vi "AlliGator Get-Set Loading & Pre-Processing Options.vi"(6 "Get (F)/Set":bool, 8 "Error In":errorcluster, 11 "Dataset Loading & Pre-processing Options (in)":T1={"Data Information"={"Gates to Skip"={"Start"=0, "End"=0}, "# Gates"=1, "Gate Step"=1, "Gate Duration"=3e-10, "Gate Separation"=4e-11, "Pile-up Correction"=FALSE, "Pixel Well Capacity"=1, "Define Gates to"=enum."Skip", "Gates to Keep"={"First"=0, "Last"=0}, "Laser Period"=0.0, "SYNC Period"=0.0, "Channel Name"=0, "Channel Arithmetic"=enum."None", "Background File Subtraction"=FALSE, "Background Scaling Factor"=1.0, "Background File"=path "", "Background Pile-up Correction"=FALSE, "Background Pixel Well Capacity"=1, "Dataset Scaling Factor"=1.0}, "Source Image Settings"={"Low Count Pixels Rejection Options"={"Background Low Threshold Factor"=0.0, "Fixed Low Background Threshold"=20000.0, "Reject Low Count Pixels"=FALSE, "Low Percentile"=0.0}, "High Count Pixels Rejection Options"={"Background High Threshold Factor"=0.0, "Fixed High Background Threshold"=1.0, "Reject High Count Pixels"=FALSE, "High Percentile"=100.0}, "Peak Threshold"=500.0, "Intensity Threshold"=500.0, "Image Smoothing Options"={"Use Image Smoothing"=FALSE, "Kernel Type"=enum."Bilinear", "Bin"=1, "Algorithm"=enum."Rapid"}, "Image Binning Options"={"Use Image Binning"=FALSE, "X Bin"=1, "Y Bin"=1}}, "Decay Preprocessing Options & Parameters"={"Background Subtraction Parameters"={"Background Definition Range"={"Min Gate"=0.0, "Max Gate"=0.0}, "Baseline Subtraction Method"=enum."Mean", "Background Subtraction?"=FALSE, "Background File"=path "", "Background Constant"=0.0, "Background Scaling Factor"=1.0, "Background Pile-up Correction"=FALSE, "Background Pixel Well Capacity"=1}, "Decay Preprocessing Parameters"={"Background Subtraction"=FALSE, "Straighten Decay"=FALSE, "Reverse Gates"=FALSE, "1-Normalized Decay"=FALSE, "Smoothen Decay"=FALSE, "Smoothing Parameter"=0.0, "Shift Decay"=FALSE, "Decay Shift Parameters"={"Type"=enum."Default", "Shift"=0.0, "Threshold"=0.0, "Rotate"=FALSE}, "Extrapolate Decay"=FALSE, "Additional Points"=0, "Head Fraction"=0.0, "Pixel-Normalize Decay"=FALSE, "Use Periodicity"=FALSE, "Use Cursors"=FALSE, "Tail Fraction"=0.0, "Use Decay Pre-Processing"=TRUE, "Fold Decay"=FALSE, "# Folds"=1, "[0-1]-Normalized Decay"=FALSE}, "Preprocessing Steps Order"=[]}, "Clear Phasor Graph"=FALSE} {"Decay Preprocessing Options & Parameters"."Decay Preprocessing Parameters"."# Folds" min=1; "Decay Preprocessing Options & Parameters"."Background Subtraction Parameters"."Background Pixel Well Capacity" min=1 step=1; "Source Image Settings"."Image Binning Options"."Y Bin" min=1; "Source Image Settings"."Image Binning Options"."X Bin" min=1; "Source Image Settings"."Image Smoothing Options"."Bin" min=1; "Source Image Settings"."High Count Pixels Rejection Options"."High Percentile" min=0.0 max=100.0; "Source Image Settings"."Low Count Pixels Rejection Options"."Low Percentile" min=0.0 max=100.0; "Data Information"."Background Pixel Well Capacity" min=1 step=1; "Data Information"."Channel Name" items=["Bottom INT Gate", "Bottom G2 Gate"]; "Data Information"."SYNC Period" min=0.0 format="%#.3g"; "Data Information"."Laser Period" min=0.0 format="%#.3g"; "Data Information"."Pixel Well Capacity" min=1 step=1; "Data Information"."# Gates" min=1 step=1; "Data Information"."Gate Step" min=1 step=1; "Data Information"."Gate Duration" min=0.0 format="%#.3g"; "Data Information"."Gate Separation" min=0.0 format="%#.3g"}) -> (0 "Error Out":errorcluster, 3 "Dataset Loading & Pre-processing Options (out)":T1={"Data Information"={"Gates to Skip"={"Start"=0, "End"=0}, "# Gates"=1, "Gate Step"=1, "Gate Duration"=3e-10, "Gate Separation"=4e-11, "Pile-up Correction"=FALSE, "Pixel Well Capacity"=1, "Define Gates to"=enum."Skip", "Gates to Keep"={"First"=0, "Last"=0}, "Laser Period"=0.0, "SYNC Period"=0.0, "Channel Name"=0, "Channel Arithmetic"=enum."None", "Background File Subtraction"=FALSE, "Background Scaling Factor"=1.0, "Background File"=path "", "Background Pile-up Correction"=FALSE, "Background Pixel Well Capacity"=1, "Dataset Scaling Factor"=1.0}, "Source Image Settings"={"Low Count Pixels Rejection Options"={"Background Low Threshold Factor"=0.0, "Fixed Low Background Threshold"=20000.0, "Reject Low Count Pixels"=FALSE, "Low Percentile"=0.0}, "High Count Pixels Rejection Options"={"Background High Threshold Factor"=0.0, "Fixed High Background Threshold"=1.0, "Reject High Count Pixels"=FALSE, "High Percentile"=100.0}, "Peak Threshold"=500.0, "Intensity Threshold"=500.0, "Image Smoothing Options"={"Use Image Smoothing"=FALSE, "Kernel Type"=enum."Bilinear", "Bin"=1, "Algorithm"=enum."Rapid"}, "Image Binning Options"={"Use Image Binning"=FALSE, "X Bin"=1, "Y Bin"=1}}, "Decay Preprocessing Options & Parameters"={"Background Subtraction Parameters"={"Background Definition Range"={"Min Gate"=0.0, "Max Gate"=0.0}, "Baseline Subtraction Method"=enum."Mean", "Background Subtraction?"=FALSE, "Background File"=path "", "Background Constant"=0.0, "Background Scaling Factor"=1.0, "Background Pile-up Correction"=FALSE, "Background Pixel Well Capacity"=1}, "Decay Preprocessing Parameters"={"Background Subtraction"=FALSE, "Straighten Decay"=FALSE, "Reverse Gates"=FALSE, "1-Normalized Decay"=FALSE, "Smoothen Decay"=FALSE, "Smoothing Parameter"=0.0, "Shift Decay"=FALSE, "Decay Shift Parameters"={"Type"=enum."Default", "Shift"=0.0, "Threshold"=0.0, "Rotate"=FALSE}, "Extrapolate Decay"=FALSE, "Additional Points"=0, "Head Fraction"=0.0, "Pixel-Normalize Decay"=FALSE, "Use Periodicity"=FALSE, "Use Cursors"=FALSE, "Tail Fraction"=0.0, "Use Decay Pre-Processing"=TRUE, "Fold Decay"=FALSE, "# Folds"=1, "[0-1]-Normalized Decay"=FALSE}, "Preprocessing Steps Order"=[]}, "Clear Phasor Graph"=FALSE} {"Decay Preprocessing Options & Parameters"."Decay Preprocessing Parameters"."# Folds" min=1; "Decay Preprocessing Options & Parameters"."Background Subtraction Parameters"."Background Pixel Well Capacity" min=1 step=1; "Source Image Settings"."Image Binning Options"."Y Bin" min=1; "Source Image Settings"."Image Binning Options"."X Bin" min=1; "Source Image Settings"."Image Smoothing Options"."Bin" min=1; "Source Image Settings"."High Count Pixels Rejection Options"."High Percentile" min=0.0 max=100.0; "Source Image Settings"."Low Count Pixels Rejection Options"."Low Percentile" min=0.0 max=100.0; "Data Information"."Background Pixel Well Capacity" min=1 step=1; "Data Information"."Channel Name" items=["Bottom INT Gate", "Bottom G2 Gate"]; "Data Information"."SYNC Period" min=0.0 format="%#.3g"; "Data Information"."Laser Period" min=0.0 format="%#.3g"; "Data Information"."Pixel Well Capacity" min=1 step=1; "Data Information"."# Gates" min=1 step=1; "Data Information"."Gate Step" min=1 step=1; "Data Information"."Gate Duration" min=0.0 format="%#.3g"; "Data Information"."Gate Separation" min=0.0 format="%#.3g"})   [LabVIEW 2021, in "AlliGator Scripts.lvlib"]
doc: "Gets/Sets <B>Data Information</B>, <B>Source Image Settings</b> and <B>Decay Preprocessing</B> from/in the Settings Storage.vi."
uses:
  AlliGator Scripts.lvlib
  AlliGator Data Load & Process Options.ctl
  AlliGator Data Information.ctl
  Settings/AlliGator Background Subtraction Parameters.ctl
  Settings/AlliGator Define Gates to.ctl
  Settings/AlliGator Gates to Keep.ctl
  Settings/AlliGator Gate Arithmetic.ctl
  AlliGator Source Image Settings.ctl
  Settings/AlliGator Low Count Pixels Rejection Options.ctl
  Settings/AlliGator High Count Pixels Rejection Options.ctl
  Settings/AlliGator Image Smoothing Options.ctl
  Arrays/Kernel Type.ctl
  Arrays/Smoothing Algorithm.ctl
  Source Image/AlliGator Image Binning Options.ctl
  Decay Analysis/Decay Preprocessing/AlliGator Decay Preprocessing Options.ctl
  Decay Analysis/Decay Preprocessing/AlliGator Background Subtraction Parameters.ctl
  Decay Analysis/Decay Preprocessing/AlliGator Baseline Subtraction Method.ctl
  Decay Analysis/Decay Preprocessing/AlliGator Decay Preprocessing Parameters.ctl
  Graphs/XY Graph/XY Graph Plot Shift Parameters.ctl
  Graphs/XY Graph/XY Graph Plot Shift Method.ctl
  Decay Analysis/Decay Preprocessing/AlliGator Decay Preprocessing.lvlib
  Graphs/XY Graph/XY Graph Add-Ons.lvlib
  Settings/AlliGator Settings.lvlib
  Arrays/Arrays.lvlib
  Source Image/AlliGator Source Image.lvlib
panel:
  # "see the AlliGator License on the block diagram (Ctrl+E or Window:Show Block Diagram)"
  # "Gates Characteristics"
  # "Background File Subtraction"
  # "Gates Characteristics"
  # "Background File Subtraction"
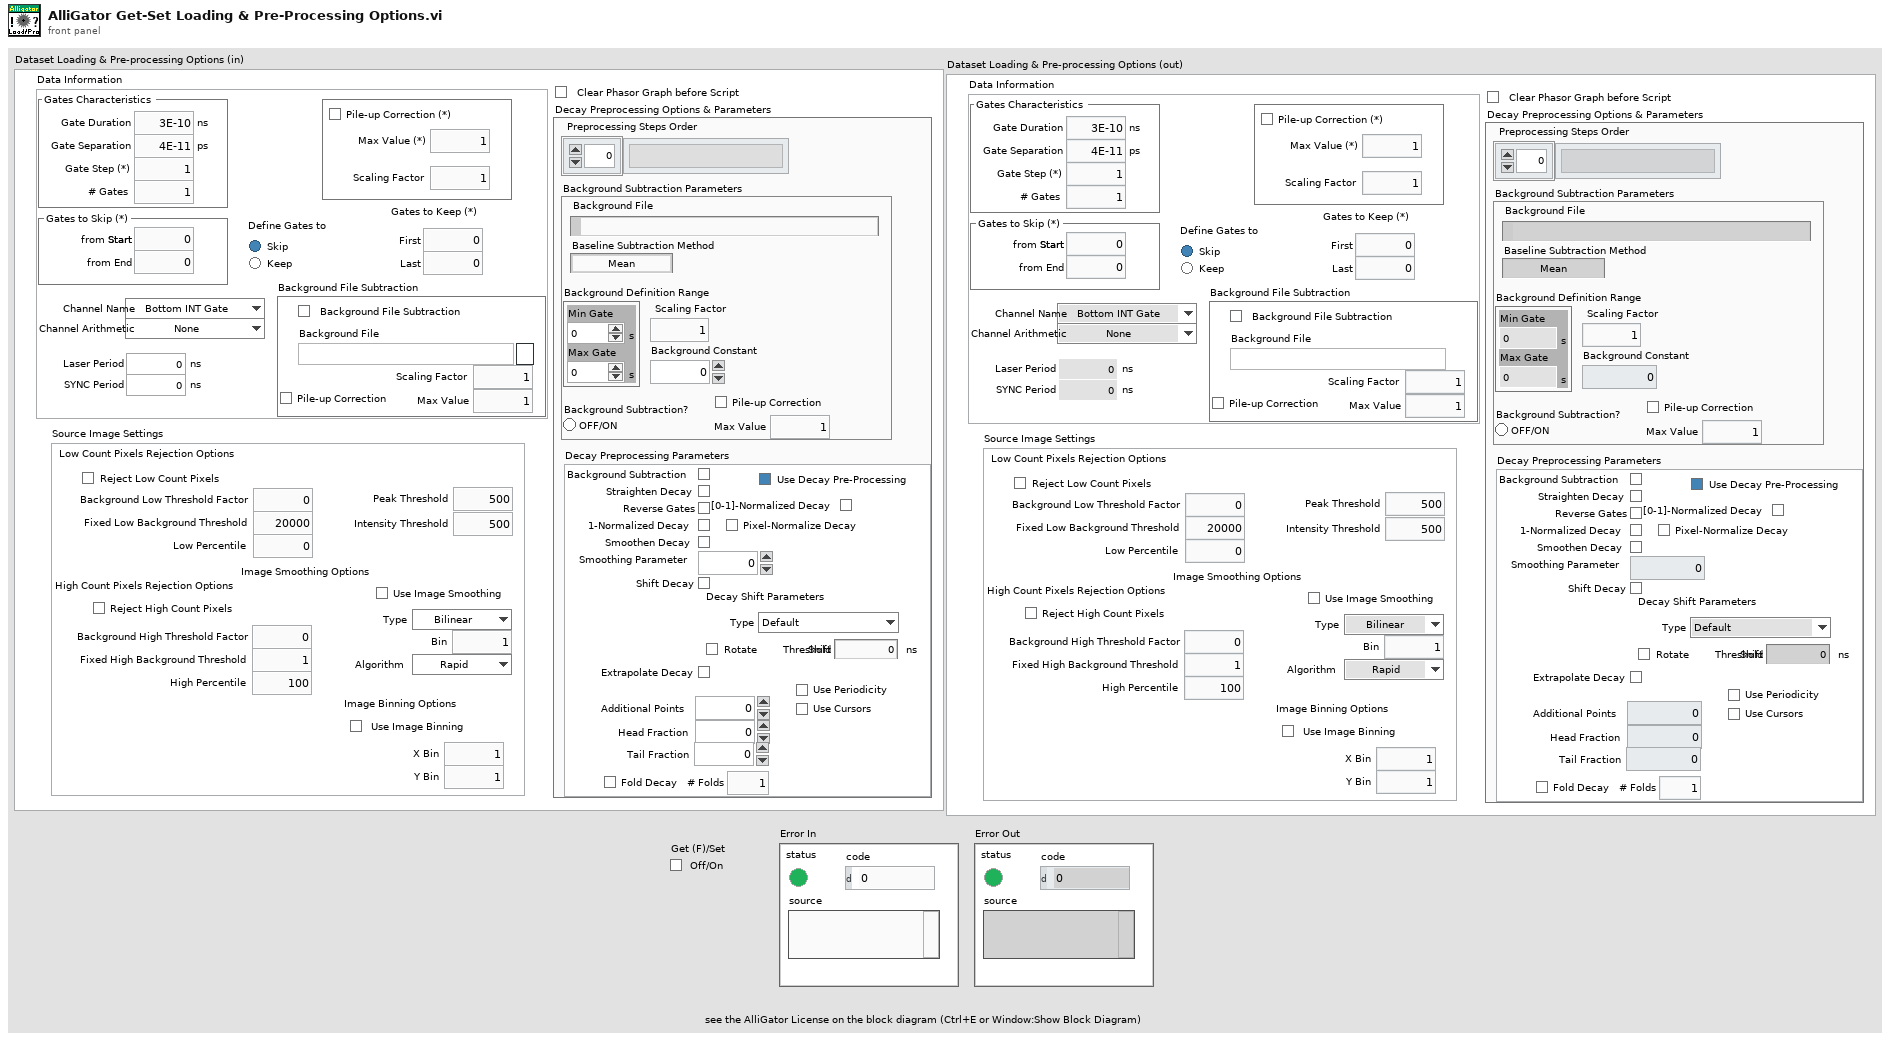
[diagram p1: front panel]
types:
  T1 = typedef "AlliGator Scripts.lvlib/AlliGator Data Load & Process Options.ctl" = cluster{"Data Information":T2, "Source Image Settings":T7, "Decay Preprocessing Options & Parameters":T14, "Clear Phasor Graph":bool}
  T2 = typedef "AlliGator Scripts.lvlib/AlliGator Data Information.ctl" = cluster{"Gates to Skip":T3, "# Gates":u32, "Gate Step":u32, "Gate Duration":dbl[unit], "Gate Separation":dbl[unit], "Pile-up Correction":bool, "Pixel Well Capacity":u32, "Define Gates to":T4, "Gates to Keep":T5, "Laser Period":dbl[unit], "SYNC Period":dbl[unit], "Channel Name":u16, "Channel Arithmetic":T6, "Background File Subtraction":bool, "Background Scaling Factor":dbl, "Background File":path, "Background Pile-up Correction":bool, "Background Pixel Well Capacity":u32, "Dataset Scaling Factor":dbl}
  T3 = typedef "AlliGator Settings.lvlib/AlliGator Background Subtraction Parameters.ctl" = cluster{"Start":u32, "End":u32}
  T4 = typedef "AlliGator Settings.lvlib/AlliGator Define Gates to.ctl" = enum32{"Skip", "Keep"}
  T5 = typedef "AlliGator Settings.lvlib/AlliGator Gates to Keep.ctl" = cluster{"First":u32, "Last":u32}
  T6 = typedef "AlliGator Settings.lvlib/AlliGator Gate Arithmetic.ctl" = enum16{"None", "INT-G2", "G2/INT*<INT>", "(1 - G2/INT)*<INT>"}
  T7 = typedef "AlliGator Scripts.lvlib/AlliGator Source Image Settings.ctl" = cluster{"Low Count Pixels Rejection Options":T8, "High Count Pixels Rejection Options":T9, "Peak Threshold":dbl, "Intensity Threshold":dbl, "Image Smoothing Options":T10, "Image Binning Options":T13}
  T8 = typedef "AlliGator Settings.lvlib/AlliGator Low Count Pixels Rejection Options.ctl" = cluster{"Background Low Threshold Factor":dbl, "Fixed Low Background Threshold":dbl, "Reject Low Count Pixels":bool, "Low Percentile":dbl}
  T9 = typedef "AlliGator Settings.lvlib/AlliGator High Count Pixels Rejection Options.ctl" = cluster{"Background High Threshold Factor":dbl, "Fixed High Background Threshold":dbl, "Reject High Count Pixels":bool, "High Percentile":dbl}
  T10 = typedef "AlliGator Settings.lvlib/AlliGator Image Smoothing Options.ctl" = cluster{"Use Image Smoothing":bool, "Kernel Type":T11, "Bin":i32, "Algorithm":T12}
  T11 = typedef "Arrays.lvlib/Kernel Type.ctl" = enum16{"Uniform", "Bilinear", "Gaussian"}
  T12 = typedef "Arrays.lvlib/Smoothing Algorithm.ctl" = enum16{"Rapid", "Thorough"}
  T13 = typedef "AlliGator Source Image.lvlib/AlliGator Image Binning Options.ctl" = cluster{"Use Image Binning":bool, "X Bin":i32, "Y Bin":i32}
  T14 = typedef "AlliGator Decay Preprocessing.lvlib/AlliGator Decay Preprocessing Options.ctl" = cluster{"Background Subtraction Parameters":T15, "Decay Preprocessing Parameters":T17, "Preprocessing Steps Order":string[]}
  T15 = typedef "AlliGator Decay Preprocessing.lvlib/AlliGator Background Subtraction Parameters.ctl" = cluster{"Background Definition Range":cluster{"Min Gate":dbl[unit], "Max Gate":dbl[unit]}, "Baseline Subtraction Method":T16, "Background Subtraction?":bool, "Background File":path, "Background Constant":dbl, "Background Scaling Factor":dbl, "Background Pile-up Correction":bool, "Background Pixel Well Capacity":u32}
  T16 = typedef "AlliGator Decay Preprocessing.lvlib/AlliGator Baseline Subtraction Method.ctl" = enum16{"Mean", "Min", "Square Gated Single-Exponential", "File", "Constant"}
  T17 = typedef "AlliGator Decay Preprocessing.lvlib/AlliGator Decay Preprocessing Parameters.ctl" = cluster{"Background Subtraction":bool, "Straighten Decay":bool, "Reverse Gates":bool, "1-Normalized Decay":bool, "Smoothen Decay":bool, "Smoothing Parameter":dbl, "Shift Decay":bool, "Decay Shift Parameters":T18, "Extrapolate Decay":bool, "Additional Points":u32, "Head Fraction":dbl, "Pixel-Normalize Decay":bool, "Use Periodicity":bool, "Use Cursors":bool, "Tail Fraction":dbl, "Use Decay Pre-Processing":bool, "Fold Decay":bool, "# Folds":u32, "[0-1]-Normalized Decay":bool}
  T18 = typedef "XY Graph Add-Ons.lvlib/XY Graph Plot Shift Parameters.ctl" = cluster{"Type":T19, "Shift":dbl[unit], "Threshold":dbl, "Rotate":bool}
  T19 = typedef "XY Graph Add-Ons.lvlib/XY Graph Plot Shift Method.ctl" = enum16{"Default", "CFD", "Threshold", "Cross-Correlation"}
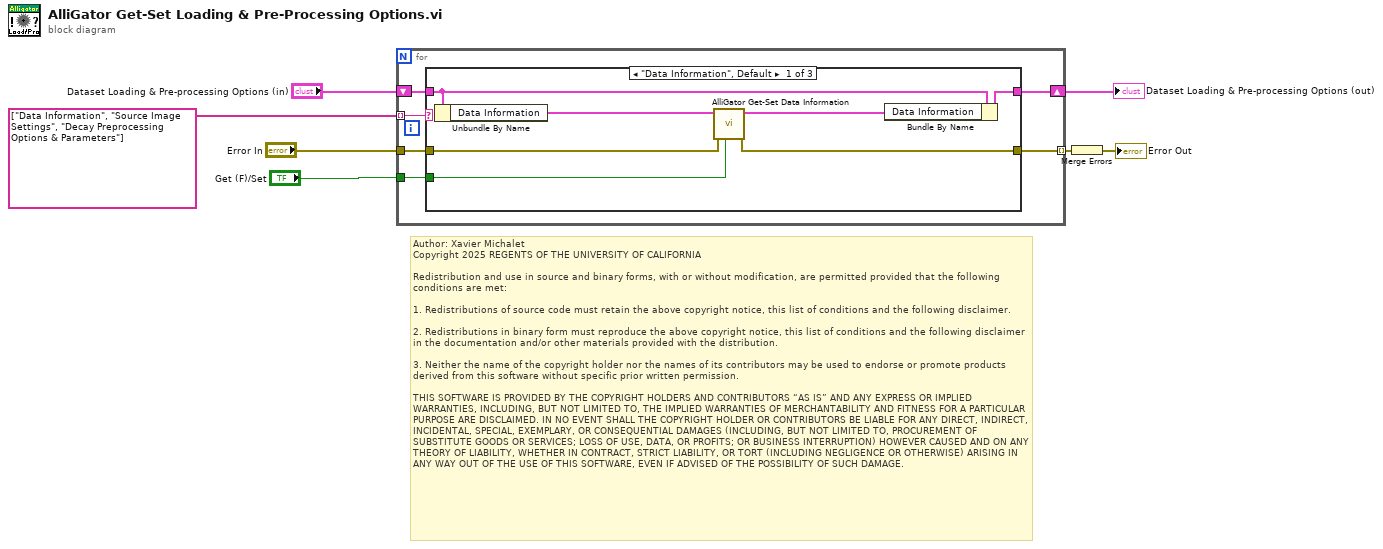
[diagram p0: block diagram]
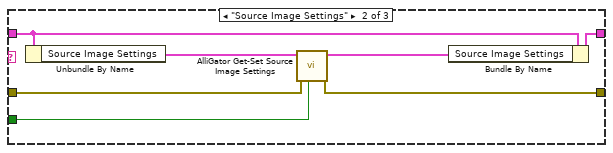
[diagram p2: hidden frame]
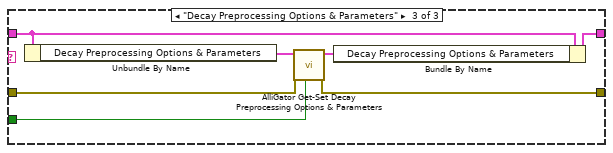
[diagram p3: hidden frame]
diagram:
  # "Author: Xavier Michalet\nCopyright 2025 REGENTS OF THE UNIVERSITY OF CALIFORNIA\n\nRedistribution and use in source and binary forms, with or without modification, are permitted provided that the following conditions are met:\n\n1. Redistributions of source code must retain the above copyright notice, this list of conditions and the following disclaimer.\n\n2. Redistributions in binary form must reproduce the above copyright notice, this list of conditions and the following disclaimer in the documentation and/or other materials provided with the distribution.\n\n3. Neither the name of the copyright holder nor the names of its contributors may be used to endorse or promote products derived from this software without specific prior written permission.\n\nTHIS SOFTWARE IS PROVIDED BY THE COPYRIGHT HOLDERS AND CONTRIBUTORS “AS IS” AND ANY EXPRESS OR IMPLIED WARRANTIES, INCLUDING, BUT NOT LIMITED TO, THE IMPLIED WARRANTIES OF MERCHANTABILITY AND FITNESS FOR A PARTICULAR PURPOSE ARE DISCLAIMED. IN NO EVENT SHALL THE COPYRIGHT HOLDER OR CONTRIBUTORS BE LIABLE FOR ANY DIRECT, INDIRECT, INCIDENTAL, SPECIAL, EXEMPLARY, OR CONSEQUENTIAL DAMAGES (INCLUDING, BUT NOT LIMITED TO, PROCUREMENT OF SUBSTITUTE GOODS OR SERVICES; LOSS OF USE, DATA, OR PROFITS; OR BUSINESS INTERRUPTION) HOWEVER CAUSED AND ON ANY THEORY OF LIABILITY, WHETHER IN CONTRACT, STRICT LIABILITY, OR TORT (INCLUDING NEGLIGENCE OR OTHERWISE) ARISING IN ANY WAY OUT OF THE USE OF THIS SOFTWARE, EVEN IF ADVISED OF THE POSSIBILITY OF SUCH DAMAGE."
  n1 = for {
    tunnel: "Get (F)/Set" -> [w13]
    shift-right: [w9] -> w3
    shift-left: "Dataset Loading & Pre-processing Options (in)" -> [w12]
    tunnel: "Error In" -> [w11]
    tunnel: [w10] -> w4 mode=indexing
    tunnel: string[] ["Data Information", "Source Image Settings", "Decay Preprocessing Options & Parameters"] -> [w8] mode=indexing
    n2 = case shown="\"Data Information\", Default" w8 {
      tunnel: w13 -> [w20 w27 w28]
      tunnel: w12 -> [w19 w26 w34]
      tunnel: w11 -> [w18 w25 w30]
      tunnel: [w17 w24 w29] -> w10
      tunnel: [w15 w22 w33] -> w9
      frame "Data Information", Default {
        n3 = Unbundle By Name(w19) -> ("Data Information"=w16:T2)
        n4 = call "AlliGator Get-Set Data Information.vi"("Get (F)/Set (T)"=w20, "error in (no error)"=w18, "Data Information in"=w16) -> ("error out"=w17:errorcluster, "Data Information out"=w14:T2)  [unwired: 7 in]
        n5 = Bundle By Name(cluster=w19, "Data Information"=w14) -> (w15:T1)
      }
      frame "Source Image Settings" {
        n6 = Unbundle By Name(w26) -> ("Source Image Settings"=w23:T7)
        n7 = call "AlliGator Get-Set Source Image Settings.vi"("Get (F)/Set (T)"=w27, "error in (no error)"=w25, "Source Image Settings in"=w23) -> ("error out"=w24:errorcluster, "Source Image Settings out"=w21:T7)  [unwired: 7 in]
        n8 = Bundle By Name(cluster=w26, "Source Image Settings"=w21) -> (w22:T1)
      }
      frame "Decay Preprocessing Options & Parameters" {
        n9 = Unbundle By Name(w34) -> ("Decay Preprocessing Options & Parameters"=w32:T14)
        n10 = call "AlliGator Get-Set Decay Preprocessing Options & Parameters.vi"("Get (F)/Set"=w28, "error in (no error)"=w30, "Decay Preprocessing Options & Parameters in"=w32) -> ("error out"=w29:errorcluster, "Decay Preprocessing Options & Parameters out"=w31:T14)  [unwired: 7 in]
        n11 = Bundle By Name(cluster=w34, "Decay Preprocessing Options & Parameters"=w31) -> (w33:T1)
      }
    }
  }
  "Dataset Loading & Pre-processing Options (out)" <- w3
  n12 = Merge Errors(w4) -> (→"Error Out":errorcluster)
